vi "TCP PXI DAQ Server.vi"(11 "Show stop":bool=TRUE) -> ()   [LabVIEW 2015]
uses:
  DAQ Engine VIs/PXI Globals.vi
panel:
  out "Error":bool
  out "TCP error":errorcluster
  out "data string":string
  out "DAQ in progress":bool
  out "Status":bool
  out "Ready":bool
  out "Busy":bool
  out "Primary":bool
  in  "stop":bool
  out "error out":errorcluster
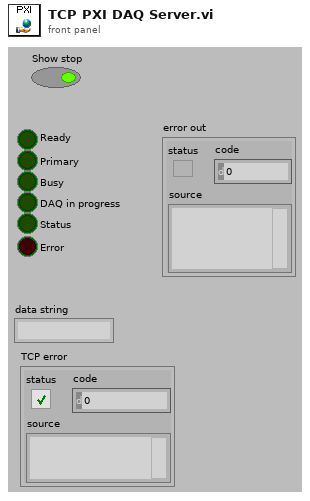
[diagram p1: front panel]
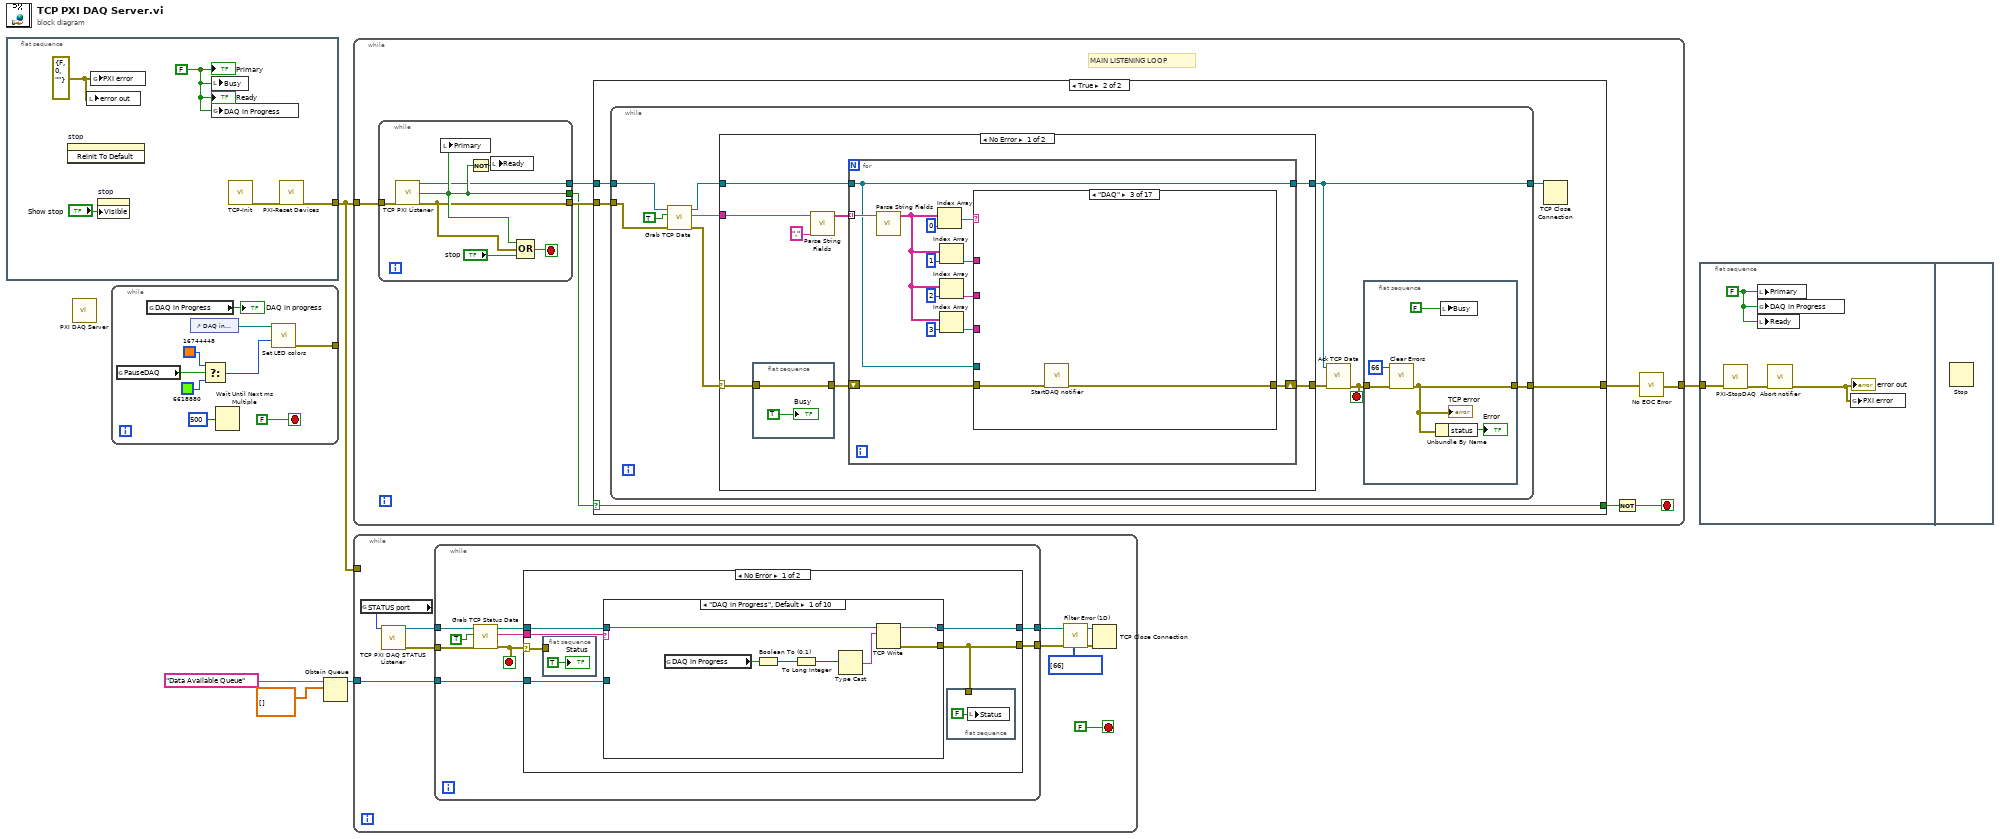
[diagram p0: block diagram]
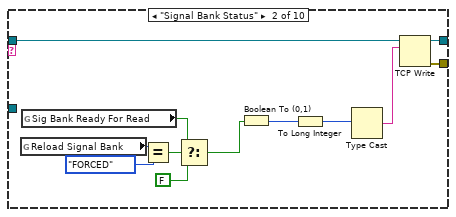
[diagram p2: hidden frame]
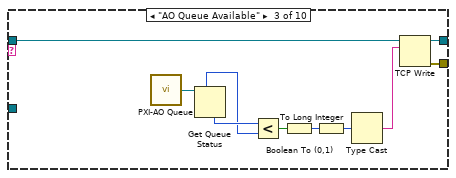
[diagram p3: hidden frame]
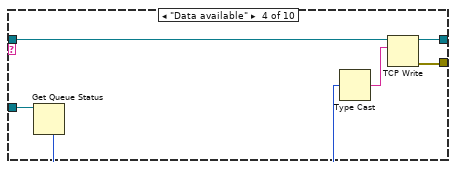
[diagram p4: hidden frame]
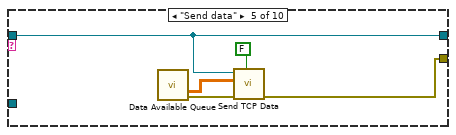
[diagram p5: hidden frame]
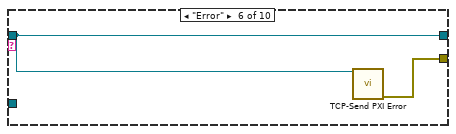
[diagram p6: hidden frame]
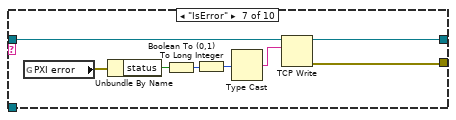
[diagram p7: hidden frame]
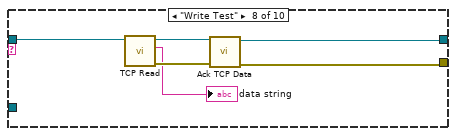
[diagram p8: hidden frame]
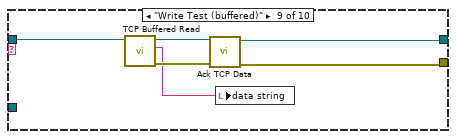
[diagram p9: hidden frame]
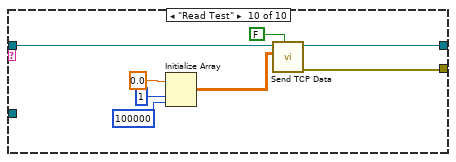
[diagram p10: hidden frame]
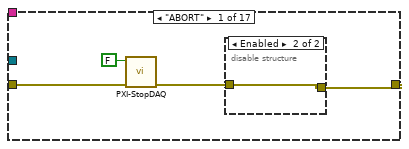
[diagram p13: hidden frame]
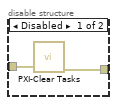
[diagram p14: hidden frame]
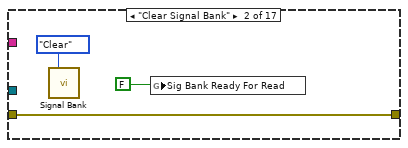
[diagram p15: hidden frame]
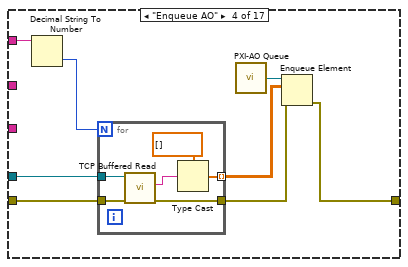
[diagram p16: hidden frame]
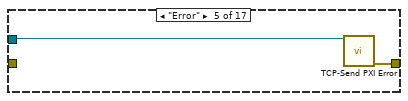
[diagram p17: hidden frame]
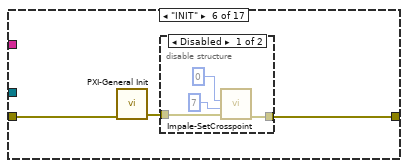
[diagram p18: hidden frame]
diagram:
  n1 = flat-sequence {
    tunnel: [w10] -> w1
    frame #0 {
      w9 = errorcluster {"status"=FALSE, "code"=0, "source"=""} ("PXI error")
      w7 = FALSE ("Connected?")
      n2 = invoke on="stop" class="Bool" method="Reinit To Default"() -> ()  [unwired: 3 in, 3 out]
      n3 = local write "error out"(w9) -> ()
      n4 = global write "PXI Globals.vi" "PXI error"(w9) -> ()
      n5 = property on="stop" class="Bool"("Visible"="Show stop") -> ()  [unwired: 2 in, 2 out]
      n6 = local write "Busy"(w7) -> ()
      n7 = global write "PXI Globals.vi" "DAQ in Progress"(w7) -> ()
      n8 = call "TCP-Init.vi"() -> ("error out"=w8:errorcluster)  [unwired: 15 in]
      n9 = call "PXI-Reset Devices.vi"("error in"=w8) -> ("error out"=w10:errorcluster)  [unwired: 10 in]
      "Primary" <- w7
      "Ready" <- w7
    }
  }
  n10 = call "PXI DAQ Server.vi"() -> ()  [unwired: 7 in, 1 out]
  n11 = while {
    tunnel: [w12] -> _
    stop <- FALSE stop-if-true
    n12 = global read "PXI Globals.vi" "PauseDAQ"() -> (w15:bool)
    n13 = global read "PXI Globals.vi" "DAQ in Progress"() -> (→"DAQ in progress":bool)
    n14 = control-ref of="DAQ in progress"() -> (w16:refnum<vi>)
    n15 = Select(t=u32 16744448, s=w15, f=u32 6618880) -> (s? t:f=w11:u32)
    n16 = Wait Until Next ms Multiple(millisecond multiple=500) -> ()  [unwired: 1 out]
    n17 = call "Set LED colors.vi"("On color"=w11, "reference"=w16) -> ("error out"=w12:errorcluster)  [unwired: 8 in, 1 out]
  }
  n18 = Obtain Queue(name (unnamed)="Data Available Queue", element data type=dbl[][] [] ("AI Waveforms 2")) -> (queue out=w2:refnum<queue>)  [unwired: 3 in, 2 out]
  n19 = while {
    tunnel: [w22] -> w5
    tunnel: w1 -> [w25]
    stop <- w21 stop-if-true
    # "MAIN LISTENING LOOP"
    n20 = while {
      tunnel: [w208] -> w27
      tunnel: w25 -> [w214]
      tunnel: [w210] -> w24
      tunnel: [w209] -> w20
      stop <- w212 stop-if-true
      n21 = call "TCP PXI Listener.vi"("error in (no error)"=w214) -> ("connection ID"=w209:refnum<k5>, "Connected?"=w210:bool, "error out"=w208:errorcluster)  [unwired: 12 in]
      n22 = local write "Primary"(w210) -> ()
      n23 = Not(x=w210) -> (.not. x?=w211:bool)
      n24 = local write "Ready"(w211) -> ()
      n25 = Compound Arithmetic op=OR(w210, w208, "stop") -> (w212:bool)
    }
    n26 = case shown="True" w24 {
      selector: w24 -> [w28 w33]
      tunnel: [w29 w32] -> w26
      tunnel: w27 -> [w29 w34]
      tunnel: [w28 w33] -> w23
      tunnel: w20 -> [_ w31]
      frame False {
      }
      frame True {
        n27 = while {
          tunnel: w34 -> [w44]
          tunnel: [w41] -> w32
          tunnel: w31 -> [w38]
          tunnel: [w36] -> w30
          stop <- w35 stop-if-true
          n28 = call "Grab TCP Data.vi"("connection ID"=w38, "No timeout?"=TRUE, "error in (no error)"=w44) -> ("connection ID 2"=w37:refnum<k5>, "data out"=w43:string, "error out"=w40:errorcluster)  [unwired: 5 in]
          n29 = case shown="No Error" w40 {
            selector: w40 -> [w52 w207]
            tunnel: [w54 w207] -> w42
            tunnel: w43 -> [w57 _]
            tunnel: w37 -> [w51 w206]
            tunnel: [w50 w206] -> w36
            frame No Error {
              n30 = flat-sequence {
                tunnel: w52 -> [w58]
                tunnel: [w58] -> w53
                frame #0 {
                  "Busy" <- TRUE ("Receiving")
                }
              }
              n31 = call "Parse String Fields.vi"("Separator"=",", "String"=w57) -> ("Fields"=w55:string[])  [unwired: 8 in, 1 out]
              n32 = for {
                tunnel: w55 -> [w61] mode=indexing
                shift-right: [w71] -> w54
                shift-left: w53 -> [w72]
                tunnel: w51 -> [w60]
                tunnel: [w60] -> w50
                n33 = call "Parse String Fields.vi"("String"=w61) -> ("Fields"=w62:string[])  [unwired: 9 in, 1 out]
                n34 = Index Array(array=w62, index=0) -> (element=w69:string)
                n35 = Index Array(array=w62, index=1) -> (element=w65:string)
                n36 = Index Array(array=w62, index=2) -> (element=w66:string)
                n37 = Index Array(array=w62, index=3) -> (element=w63:string)
                n38 = case shown="\"DAQ\"" w69 {
                  selector: w69 -> [_ _ _ _ _ _ _ _ _ _ _ _ _ _ _ _ w198]
                  tunnel: w72 -> [w75 w82 w83 w89 _ w101 w109 w113 w117 w123 w143 w153 w158 w161 w183 w196 w204]
                  tunnel: [w76 w82 w84 w91 w100 w103 w109 w113 w116 w124 w140 w153 w155 w163 w182 w196 w197] -> w71
                  tunnel: w66 -> [_ _ _ _ _ _ _ _ w115 w121 _ _ w157 w160 w181 _ _]
                  tunnel: w65 -> [_ _ _ w86 _ _ _ w111 _ _ _ _ _ w162 _ _ _]
                  tunnel: w63 -> [_ _ _ _ _ _ _ _ w114 w118 w141 _ w156 w159 _ _ _]
                  tunnel: w60 -> [_ _ _ w90 w99 _ _ _ _ w119 w142 _ _ _ _ _ _]
                  frame "ABORT" {
                    n39 = call "PXI-StopDAQ.vi"("error in (no error)"=w75, "Wait for DAQ to stop? (T)"=FALSE) -> ("error out"=w74:errorcluster)  [unwired: 5 in]
                    n40 = disable-structure shown="Enabled" {
                      disable-tunnel: w74 -> [w78 w79]
                      disable-tunnel: [w77 w79] -> w76
                      frame Disabled {
                        n41 = call "PXI-Clear Tasks.vi"("error in (no error)"=w78) -> ("error out"=w77:errorcluster)  [unwired: 14 in]
                      }
                      frame Enabled {
                      }
                    }
                  }
                  frame "Clear Signal Bank" {
                    n42 = call "Signal Bank.vi"("Action"=enum16{"Add", "Replace ID", "Read ID", "Clear"}."Clear") -> ()  [unwired: 13 in, 2 out]
                    n43 = global write "PXI Globals.vi" "Sig Bank Ready For Read"(FALSE ("DAQ Connected")) -> ()
                  }
                  frame "DAQ" {
                    n44 = call "StartDAQ notifier.vi"("error in (no error)"=w83) -> ("error out"=w84:errorcluster)  [unwired: 6 in]
                  }
                  frame "Enqueue AO" {
                    n45 = Decimal String To Number(string=w86) -> (number=w85:i32)  [unwired: 2 in, 1 out]
                    n46 = for {
                      N: w85 -> [_]
                      tunnel: w90 -> [w98]
                      tunnel: w89 -> [w97]
                      tunnel: [w94] -> w87 mode=indexing
                      tunnel: [w93] -> w88
                      n47 = call "TCP Buffered Read.vi"("error in (no error)"=w97, "connection ID"=w98) -> ("error out"=w93:errorcluster, "data string"=w95:string)  [unwired: 6 in, 2 out]
                      n48 = Type Cast(type=dbl[] [], x=w95) -> (*(type *) &x=w94:dbl[])
                    }
                    n49 = call "PXI-AO Queue.vi"() -> ("Queue"=w92:refnum<queue>)  [unwired: 15 in]
                    n50 = Enqueue Element(queue=w92, element=w87, error in (no error)=w88) -> (error out=w91:errorcluster)  [unwired: 1 in, 2 out]
                  }
                  frame "Error" {
                    n51 = call "TCP-Send PXI Error.vi"("connection ID"=w99) -> ("error out"=w100:errorcluster)  [unwired: 14 in]
                  }
                  frame "INIT" {
                    n52 = call "PXI-General Init.vi"("error in (no error)"=w101) -> ("error out"=w102:errorcluster)  [unwired: 10 in]
                    n53 = disable-structure shown="Disabled" {
                      disable-tunnel: [w107 w108] -> w103
                      disable-tunnel: w102 -> [w104 w108]
                      frame Disabled {
                        n54 = call "Impale-SetCrosspoint.vi"("error in (no error)"=w104, "Site"=7, "Bank"=0) -> ("error out"=w107:errorcluster)  [unwired: 4 in]
                      }
                      frame Enabled {
                      }
                    }
                  }
                  frame "NOOP" {
                    # "// do nothing"
                  }
                  frame "Pause" {
                    n55 = Decimal String To Number(string=w111) -> (number=w112:i32)  [unwired: 2 in, 1 out]
                    n56 = Not Equal To 0?(x=w112) -> (x != 0?=w110:bool)
                    n57 = global write "PXI Globals.vi" "PauseDAQ"(w110) -> ()
                  }
                  frame "SETKEY" {
                    n58 = call "TCP-Parse Key.vi"("error in (no error)"=w117, "Value"=w114, "Key"=w115) -> ("error out"=w116:errorcluster)  [unwired: 8 in]
                  }
                  frame "SETWAVE" {
                    n59 = case shown="\"BUF\"" w118 {
                      tunnel: w123 -> [w128 w132]
                      tunnel: [w127 w131] -> w122
                      tunnel: [w126 w130] -> w120
                      tunnel: w119 -> [w125 w129]
                      frame "BUF" {
                        n60 = call "TCP Buffered Read.vi"("error in (no error)"=w128, "connection ID"=w125) -> ("error out"=w126:errorcluster, "data string"=w127:string)  [unwired: 6 in, 2 out]
                      }
                      frame "UNBUF", Default {
                        n61 = call "TCP Read.vi"("error in (no error)"=w132, "connection ID"=w129) -> ("error out"=w130:errorcluster, "data string"=w131:string)  [unwired: 7 in, 1 out]
                      }
                    }
                    n62 = case shown="No Error" w120 {
                      selector: w120 -> [w133 w139]
                      tunnel: [w133 w139] -> w124
                      tunnel: w122 -> [w137 _]
                      tunnel: w121 -> [w134 _]
                      frame No Error {
                        # "all WAVEs are assumed\nto be binary DOUBLEs"
                        n63 = Type Cast(type=dbl[] [], x=w137) -> (*(type *) &x=w135:dbl[])
                        n64 = call "Signal Bank.vi"("Action"=enum16{"Add", "Replace ID", "Read ID", "Clear"}."Add", "1D Data In"=w135, "ID"=w134) -> ()  [unwired: 11 in, 2 out]
                      }
                      frame Error {
                      }
                    }
                  }
                  frame "BufferedWriteTest" {
                    n65 = case shown="\"BUF\"" w141 {
                      tunnel: w143 -> [w148 w152]
                      tunnel: [w147 w151] -> _
                      tunnel: [w146 w150] -> w140
                      tunnel: w142 -> [w145 w149]
                      frame "BUF" {
                        n66 = call "TCP Buffered Read.vi"("error in (no error)"=w148, "timeout (ms)"=1000, "connection ID"=w145) -> ("error out"=w146:errorcluster, "data string"=w147:string)  [unwired: 5 in, 2 out]
                      }
                      frame "UNBUF", Default {
                        n67 = call "TCP Read.vi"("error in (no error)"=w152, "connection ID"=w149) -> ("error out"=w150:errorcluster, "data string"=w151:string)  [unwired: 7 in, 1 out]
                      }
                    }
                  }
                  frame "STOPDAQ" {
                    n68 = global write "PXI Globals.vi" "StopDAQ"(TRUE) -> ()
                  }
                  frame "Set Multipliers" {
                    n69 = call "TCP-Set AO Gains.vi"("error in (no error)"=w158, "Gain String"=w156, "Channel String"=w157) -> ("error out"=w155:errorcluster)  [unwired: 8 in]
                  }
                  frame "SetAOGains" {
                    n70 = case shown="No Error" w161 {
                      selector: w161 -> [w169 w173]
                      tunnel: [w166 w173] -> w163
                      tunnel: w162 -> [w167 _]
                      tunnel: w160 -> [w165 _]
                      tunnel: w159 -> [w164 _]
                      frame No Error {
                        n71 = call "TCP-Set AO Gains.vi"("error in (no error)"=w169, "Gain String"=w164, "Channel String"=w165) -> ("error out"=w168:errorcluster)  [unwired: 8 in]
                        n72 = case shown="\"OTF\"" w167 {
                          tunnel: w168 -> [w170 w172]
                          tunnel: [w170 w171] -> w166
                          frame "False", Default {
                          }
                          frame "OTF" {
                            n73 = call "PXI-Set AO Gains OTF.vi"("error in (no error)"=w172) -> ("error out"=w171:errorcluster)  [unwired: 10 in]
                          }
                        }
                      }
                      frame Error {
                      }
                    }
                  }
                  frame "TRIG" {
                    n74 = Obtain Notifier(name (unnamed)=w181, notification data type=FALSE, error in (no error)=w183) -> (notifier out=w179:refnum<notifier>, error out=w178:errorcluster)  [unwired: 1 in, 1 out]
                    n75 = Get Notifier Status(notifier=w179, error in (no error)=w178) -> (notifier out=w175:refnum<notifier>, # waiting=w177:i32, error out=w174:errorcluster)  [unwired: 2 out]
                    n76 = Greater Than 0?(x=w177) -> (x > 0?=w176:bool)
                    n77 = case shown="True" w176 {
                      tunnel: [w184 w193] -> w182
                      tunnel: w175 -> [w186 w190]
                      tunnel: w174 -> [w185 w189]
                      tunnel: w181 -> [_ w188]
                      frame False {
                        # "// no one is waiting\n// on this trigger,\n// so ignore it"
                        n78 = Release Notifier(notifier=w186, force destroy? (F)=TRUE, error in (no error)=w185) -> (error out=w184:errorcluster)  [unwired: 2 out]
                      }
                      frame True {
                        n79 = case shown="\"StartDAQ\"" w188 {
                          frame Default {
                          }
                          frame "StartDAQ" {
                            # "Set DAQ in Progress here to make sure it's set for next call to  TCP Grab"
                            n80 = global write "PXI Globals.vi" "DAQ in Progress"(TRUE ("DAQ in Progress")) -> ()
                          }
                        }
                        n81 = Unbundle By Name(w189) -> ("status"=w192:bool)
                        n82 = Not(x=w192) -> (.not. x?=w191:bool)
                        n83 = Send Notification(notification=w191, notifier=w190, error in (no error)=w189) -> (error out=w193:errorcluster)  [unwired: 1 out]
                      }
                    }
                  }
                  frame "WAVEREADY" {
                    n84 = global write "PXI Globals.vi" "Sig Bank Ready For Read"(TRUE) -> ()
                  }
                  frame Default {
                    w203 = 1 items=["No error", "Argument error", "Memory is full", "Out of zone", "End of file", "File already open", "Generic file I/O error", "File not found", "File permission error", "Disk is full", "Duplicate path", "Too many files open", "System feature not enabled", "Resource file not found", "Cannot add resource", "Resource not found", "Image not found", "Image memory error", "Pen does not exist", "Config type invalid", "Config token not found", "Config parse error", "Config memory error", "Bad external code format", "Bad external code offset", "External code not present", "Null window", "Destroy window error", "Null menu", "Print aborted", "Bad print record", "Print driver error", "Windows error during printing", "Memory error during printing", "Print dialog error", "Generic print error", "Invalid device refnum", "Device not found", "Device parameter error", "Device unit error", "Cannot open device", "Device call aborted", "Generic error", "Cancelled by user", "Object ID too low", "Object ID too high", "Object not in heap", "Unknown heap", "Unknown object (invalid DefProc)", "Unknown object (DefProc not in table)", "Message out of range", "Invalid (null) method", "Unknown message", "Manager call not supported", "Bad address", "Network operation in progress", "Network operation timed out", "Connection is busy", "Network attribute not supported", "Network error", "Address in use", "System out of memory", "Connection aborted", "Connection refused", "Not connected", "Already connected", "Connection closed", "Initialization error (interapplication manager)", "Bad occurrence", "Wait on unbound occurrence handler", "Occurrence queue overflow", "Datalog type conflict", "Unused", "Unrecognized type (interapplication manager)", "Memory corrupt", "Failed to make temporary DLL", "Old CIN version", "Drag socket not found", "Failed to load drop-object", "Failed to register OLE object", "Failed to release OLE object", "Format specifier type mismatch", "Unknown format specifier", "Too few format specifiers", "Too many format specifiers", "Scan failed", "Newer CIN version", "Error converting to variant", "Runtime menu error", "Password tampered", "Variant attribute not found", "Incompatible variant data type", "Event data is not available", "Event Store is not present", "Occurrence is not found", "Event Queue is not created", "Event info is not available", "Refnum passed is NULL", "Error retrieving Class GUID", "Error retrieving CoClass GUID", "Error retrieving TypeLib GUID.", "Bad built application magic bytes.", "Specific driver is different from the specific driver associated with the Logical Name.", "There is no session opened to the class driver.", "Max Error", "MAX - Error with config objects", "MAX - Error loading configuration", "MAX - Group not supported"]
                    n85 = Current VI's Path() -> (path=w201:path)
                    n86 = Strip Path(path=w201) -> (name=w200:string)  [unwired: 1 out]
                    n87 = Format Into String(format string="%s: unrecognized TCP tag '%s'", w200, w198) -> (resulting string=w205:string)  [unwired: 2 in, 1 out]
                    n88 = Bundle By Name(cluster=w204, "code"=w203, "status"=TRUE, "source"=w205) -> (w197:errorcluster)
                  }
                }
              }
            }
            frame Error {
            }
          }
          n89 = call "Ack TCP Data.vi"("connection ID"=w36, "error in (no error)"=w42) -> ("error out"=w35:errorcluster)  [unwired: 7 in, 1 out]
          n90 = flat-sequence {
            tunnel: w35 -> [w47]
            tunnel: [w46] -> w41
            frame #0 {
              n91 = call <vilib>:"Clear Errors.vi"("error in (no error)"=w47, "specific error code to clear (0: all)"=66) -> ("error out"=w46:errorcluster)  [unwired: 4 in, 1 out]
              "TCP error" <- w46
              n92 = Unbundle By Name(w46) -> ("status"=→"Error":bool)
              n93 = local write "Busy"(FALSE ("Receiving")) -> ()
            }
          }
        }
        n94 = TCP Close Connection(connection ID=w30) -> ()  [unwired: 2 in, 2 out]
      }
    }
    n95 = Not(x=w23) -> (.not. x?=w21:bool)
    n96 = call "No EOC Error.vi"("error in"=w26) -> ("error out"=w22:errorcluster)  [unwired: 4 in]
  }
  n97 = while {
    tunnel: w2 -> [w220]
    tunnel: w1 -> [_]
    stop <- FALSE stop-if-true
    n98 = global read "PXI Globals.vi" "STATUS port"() -> (w221:u16)
    n99 = call "TCP PXI DAQ STATUS Listener.vi"("port"=w221) -> ("connection ID"=w219:refnum<k5>, "error out"=w223:errorcluster)  [unwired: 12 in, 1 out]
    n100 = while {
      tunnel: w223 -> [w231]
      tunnel: [w230] -> w218
      tunnel: w220 -> [w229]
      tunnel: w219 -> [w227]
      tunnel: [w224] -> w217
      stop <- w225 stop-if-true
      n101 = call "Grab TCP Status Data.vi"("connection ID"=w227, "No timeout?"=TRUE, "error in (no error)"=w231) -> ("Status ID out"=w226:refnum<k5>, "data out"=w232:string, "error out"=w225:errorcluster)  [unwired: 5 in]
      n102 = case shown="No Error" w225 {
        selector: w225 -> [w233 w312]
        tunnel: w232 -> [w238 _]
        tunnel: [w234 w312] -> w230
        tunnel: w229 -> [w237 _]
        tunnel: w226 -> [w236 w311]
        tunnel: [w235 w311] -> w224
        frame No Error {
          n103 = flat-sequence {
            tunnel: w233 -> [_]
            frame #0 {
              "Status" <- TRUE ("Status")
            }
          }
          n104 = case shown="\"DAQ in Progress\", Default" w238 {
            tunnel: [w244 w256 w268 w274 w277 w282 w285 w293 w302 w303] -> w234
            tunnel: w237 -> [_ _ _ w273 _ _ _ _ _ _]
            tunnel: w236 -> [w242 w249 w267 w271 w276 w281 w284 w296 w300 w310]
            tunnel: [w241 w248 w266 w270 w276 w281 w283 w292 w301 w309] -> w235
            frame "DAQ in Progress", Default {
              n105 = global read "PXI Globals.vi" "DAQ in Progress"() -> (w243:bool)
              n106 = Boolean To (0,1)(Boolean=w243) -> (0, 1=w246:i16)
              n107 = To Long Integer(number=w246) -> (32bit integer=w245:i32)
              n108 = Type Cast(x=w245) -> (*(type *) &x=w247:string)  [unwired: 1 in]
              n109 = TCP Write(connection ID=w242, data in=w247) -> (connection ID out=w241:refnum<k5>, error out=w244:errorcluster)  [unwired: 2 in, 1 out]
            }
            frame "Signal Bank Status" {
              n110 = global read "PXI Globals.vi" "Reload Signal Bank"() -> (w255:enum32{"OFF", "ENABLED", "FORCED"})
              n111 = global read "PXI Globals.vi" "Sig Bank Ready For Read"() -> (w252:bool)
              n112 = Equal?(x=w255, y=enum32{"OFF", "ENABLED", "FORCED"}."FORCED") -> (x = y?=w253:bool)
              n113 = Select(t=w252, s=w253, f=FALSE) -> (s? t:f=w250:bool)
              n114 = Boolean To (0,1)(Boolean=w250) -> (0, 1=w258:i16)
              n115 = To Long Integer(number=w258) -> (32bit integer=w257:i32)
              n116 = Type Cast(x=w257) -> (*(type *) &x=w259:string)  [unwired: 1 in]
              n117 = TCP Write(connection ID=w249, data in=w259) -> (connection ID out=w248:refnum<k5>, error out=w256:errorcluster)  [unwired: 2 in, 1 out]
            }
            frame "AO Queue Available" {
              n118 = call "PXI-AO Queue.vi"() -> ("Queue"=w265:refnum<queue>)  [unwired: 15 in]
              n119 = Get Queue Status(queue=w265) -> (max queue size=w263:i32, # elements in queue=w264:i32)  [unwired: 2 in, 6 out]
              n120 = Less?(x=w264, y=w263) -> (x < y?=w262:bool)
              n121 = Boolean To (0,1)(Boolean=w262) -> (0, 1=w261:i16)
              n122 = To Long Integer(number=w261) -> (32bit integer=w260:i32)
              n123 = Type Cast(x=w260) -> (*(type *) &x=w269:string)  [unwired: 1 in]
              n124 = TCP Write(connection ID=w267, data in=w269) -> (connection ID out=w266:refnum<k5>, error out=w268:errorcluster)  [unwired: 2 in, 1 out]
            }
            frame "Data available" {
              n125 = Get Queue Status(queue=w273) -> (# elements in queue=w272:i32)  [unwired: 2 in, 7 out]
              n126 = Type Cast(x=w272) -> (*(type *) &x=w275:string)  [unwired: 1 in]
              n127 = TCP Write(connection ID=w271, data in=w275) -> (connection ID out=w270:refnum<k5>, error out=w274:errorcluster)  [unwired: 2 in, 1 out]
            }
            frame "Send data" {
              n128 = call "Data Available Queue.vi"() -> ("AI Waveforms"=w279:dbl[][], "error out"=w278:errorcluster)  [unwired: 11 in, 3 out]
              n129 = call "Send TCP Data.vi"("connection ID"=w276, "Data in"=w279, "error in (no error)"=w278, "Single precision?"=FALSE) -> ("error out"=w277:errorcluster)  [unwired: 5 in, 1 out]
            }
            frame "Error" {
              n130 = call "TCP-Send PXI Error.vi"("connection ID"=w281) -> ("error out"=w282:errorcluster)  [unwired: 14 in]
            }
            frame "IsError" {
              n131 = global read "PXI Globals.vi" "PXI error"() -> (w289:errorcluster)
              n132 = Unbundle By Name(w289) -> ("status"=w288:bool)
              n133 = Boolean To (0,1)(Boolean=w288) -> (0, 1=w287:i16)
              n134 = To Long Integer(number=w287) -> (32bit integer=w286:i32)
              n135 = Type Cast(x=w286) -> (*(type *) &x=w290:string)  [unwired: 1 in]
              n136 = TCP Write(connection ID=w284, data in=w290) -> (connection ID out=w283:refnum<k5>, error out=w285:errorcluster)  [unwired: 2 in, 1 out]
            }
            frame "Write Test" {
              n137 = call "TCP Read.vi"("connection ID"=w296) -> ("error out"=w294:errorcluster, "data string"=→"data string":string, "connection ID 2"=w295:refnum<k5>)  [unwired: 8 in]
              n138 = call "Ack TCP Data.vi"("connection ID"=w295, "error in (no error)"=w294) -> ("connection ID out"=w292:refnum<k5>, "error out"=w293:errorcluster)  [unwired: 7 in]
            }
            frame "Write Test (buffered)" {
              n139 = call "TCP Buffered Read.vi"("connection ID"=w300) -> ("error out"=w298:errorcluster, "data string"=w297:string, "connection ID 2"=w299:refnum<k5>)  [unwired: 7 in, 1 out]
              n140 = call "Ack TCP Data.vi"("connection ID"=w299, "error in (no error)"=w298) -> ("connection ID out"=w301:refnum<k5>, "error out"=w302:errorcluster)  [unwired: 7 in]
              n141 = local write "data string"(w297) -> ()
            }
            frame "Read Test" {
              n142 = Initialize Array(0.0 ("element"), 1 ("dimension size"), 100000 ("dimension size")) -> (w304:dbl[][])
              n143 = call "Send TCP Data.vi"("connection ID"=w310, "Data in"=w304, "Single precision?"=FALSE) -> ("connection ID 2"=w309:refnum<k5>, "error out"=w303:errorcluster)  [unwired: 6 in]
            }
          }
          n144 = flat-sequence {
            tunnel: w234 -> [_]
            frame #0 {
              n145 = local write "Status"(FALSE ("Status")) -> ()
            }
          }
        }
        frame Error {
        }
      }
    }
    n146 = call "Filter Error (1D).vi"("error in (no error)"=w218, "Array"=i32[] [66]) -> ("error out"=w216:errorcluster)  [unwired: 9 in]
    n147 = TCP Close Connection(connection ID=w217, error in (no error)=w216) -> ()  [unwired: 1 in, 2 out]
  }
  n148 = flat-sequence {
    tunnel: w5 -> [w315]
    frame #0 {
      w316 = FALSE ("DAQ in Progress")
      n149 = call "PXI-StopDAQ.vi"("error in (no error)"=w315) -> ("error out"=w314:errorcluster)  [unwired: 6 in]
      n150 = local write "Primary"(w316) -> ()
      n151 = global write "PXI Globals.vi" "DAQ in Progress"(w316) -> ()
      n152 = local write "Ready"(w316) -> ()
      n153 = call "Abort notifier.vi"("error in (no error)"=w314) -> ("error out"=w313:errorcluster)  [unwired: 5 in, 1 out]
      "error out" <- w313
      n154 = global write "PXI Globals.vi" "PXI error"(w313) -> ()
    }
    frame #1 {
      n155 = Stop() -> ()  [unwired: 1 in]
    }
  }
